vi "SentinelController v33.vi"() -> ()   [LabVIEW 2011] (continued)
                                n3052 = local read "GPIB wait timeout hid"() -> (w2476:u32)
                                n3053 = VISA Open(timeout (0)=w2475, VISA resource name=w2477) -> (VISA resource name=w2474:refnum<visa-resource-name>, error out=w2479:errorcluster)  [unwired: 3 in]
                                n3054 = property class="GPIB Instr"(reference=w2474, error in=w2479, "Timeout"=w2476) -> (error out=w2473:errorcluster)  [unwired: 1 out]
                                n3055 = local write "VISA bus 2 resource name out hid"(w2474) -> ()
                                n3056 = Unbundle By Name(w2473) -> ("status"=w2478:bool)
                                n3057 = local write "VISA bus 2 error out hid"(w2473) -> ()
                                n3058 = local write "VISA bus 2 open error"(w2478) -> ()
                                }
                                frame #1 {
                                n3059 = local write "Exit SC tester H2 StMach hid"(FALSE ("Exit H2 state machine hid")) -> ()
                                n3060 = Concatenate Strings("Bus 2 initializing" ("string"), "\r\n") -> (w2482:string)
                                n3061 = local write "GPIB bus 2 traffic"(w2482) -> ()
                                }
                                frame #2 {
                                n3062 = local write "MT99XX tester states H2 hid"(SC_MT99XX_tester_states."sending *IDN?" ("SC virtual tester states")) -> ()
                                }
                                }
                                }
                                frame "sending *IDN?" {
                                n3063 = flat-sequence {
                                tunnel: [w2494] -> w2487
                                tunnel: [w2493] -> w2486
                                tunnel: w2487 -> [w2508]
                                tunnel: w2486 -> [w2507]
                                tunnel: [w2498] -> w2485
                                tunnel: w2485 -> [w2509]
                                frame #0 {
                                w2488 = "*IDN?"
                                n3064 = local read "VISA bus 2 resource name out hid"() -> (w2497:refnum<visa-resource-name>)
                                n3065 = local read "GPIB bus 2 traffic"() -> (w2492:string)
                                n3066 = local read "VISA bus 2 error out hid"() -> (w2496:errorcluster)
                                n3067 = Concatenate Strings(w2492, "\r\n", "Bus 2 write: " ("string"), w2488) -> (w2490:string)
                                n3068 = VISA Write(VISA resource name=w2497, write buffer=w2488, error in (no error)=w2496) -> (VISA resource name out=w2494:refnum<visa-resource-name>, error out=w2493:errorcluster)  [unwired: 1 out]
                                n3069 = local write "GPIB bus 2 traffic"(w2490) -> ()
                                n3070 = Unbundle By Name(w2493) -> ("status"=w2495:bool)
                                n3071 = local write "GPIB bus 2 write error"(w2495) -> ()
                                }
                                frame #1 {
                                n3072 = local read "GPIB bus 2 traffic"() -> (w2500:string)
                                n3073 = VISA Read(VISA resource name=w2508, byte count=u32 256, error in (no error)=w2507) -> (VISA resource name out=w2505:refnum<visa-resource-name>, read buffer=w2499:string, error out=w2504:errorcluster)  [unwired: 1 out]
                                n3074 = local write "VISA bus 2 resource name out hid"(w2505) -> ()
                                n3075 = Unbundle By Name(w2504) -> ("status"=w2498:bool)
                                n3076 = local write "H2 response to *IDN? hid"(w2499) -> ()
                                n3077 = local write "GPIB bus 2 read error"(w2498) -> ()
                                n3078 = Concatenate Strings(w2500, "\r\n", "Bus 2 read: " ("string"), w2499) -> (w2502:string)
                                n3079 = local write "GPIB bus 2 traffic"(w2502) -> ()
                                }
                                frame #2 {
                                n3080 = case shown="True" w2509 {
                                frame False {
                                n3081 = local write "MT99XX tester states H2 hid"(SC_MT99XX_tester_states."polling *SITES?" ("SC virtual tester states")) -> ()
                                }
                                frame True {
                                n3082 = flat-sequence {
                                frame #0 {
                                n3083 = while {
                                stop <- w2512 stop-if-true
                                n3084 = One Button Dialog(message="Warning:\nVirtual tester does not get a response\nto *IDN? from handler 2.\nCheck GPIB cable and that  handler 2 \nis running and ready to issue a start of test\nby responding with sites ready.", button name ("OK")="Dismiss and retry") -> (true=w2512:bool)
                                n3085 = Wait (ms)(milliseconds to wait=u32 100) -> ()  [unwired: 1 out]
                                }
                                }
                                frame #1 {
                                n3086 = local write "H2 online"(FALSE ("H2 online")) -> ()
                                }
                                frame #2 {
                                n3087 = local write "MT99XX tester states H2 hid"(SC_MT99XX_tester_states."sending *IDN?" ("SC virtual tester states")) -> ()
                                }
                                }
                                }
                                }
                                }
                                }
                                }
                                frame "polling *SITES?" {
                                n3088 = flat-sequence {
                                tunnel: [w2520] -> w2518
                                tunnel: [w2519] -> w2517
                                tunnel: w2518 -> [w2556]
                                tunnel: w2517 -> [w2555]
                                frame #0 {
                                n3089 = while {
                                tunnel: [w2524] -> w2520
                                tunnel: [w2521] -> w2519
                                stop <- w2523 stop-if-true
                                n3090 = stacked-sequence {
                                tunnel: [w2536] -> w2526
                                tunnel: [w2535] -> w2525
                                frame #0 {
                                w2531 = "*SITES?"
                                n3091 = local read "VISA bus 2 resource name out hid"() -> (w2528:refnum<visa-resource-name>)
                                n3092 = local read "VISA bus 2 error out hid"() -> (w2527:errorcluster)
                                n3093 = Concatenate Strings("Handler 2 cycle start" ("string"), "\r\n", "Bus 2 write: " ("string"), w2531) -> (w2533:string)
                                n3094 = VISA Write(VISA resource name=w2528, write buffer=w2531, error in (no error)=w2527) -> (VISA resource name out=w2536:refnum<visa-resource-name>, error out=w2535:errorcluster)  [unwired: 1 out]
                                n3095 = Unbundle By Name(w2535) -> ("status"=w2529:bool)
                                n3096 = local write "GPIB bus 2 traffic"(w2533) -> ()
                                n3097 = local write "GPIB bus 2 write error"(w2529) -> ()
                                }
                                }
                                n3098 = Wait (ms)(milliseconds to wait=u32 1) -> ()  [unwired: 1 out]
                                n3099 = flat-sequence {
                                tunnel: w2526 -> [w2554]
                                tunnel: w2525 -> [w2553]
                                tunnel: [w2540] -> w2524
                                tunnel: [w2538] -> w2523
                                tunnel: [w2537] -> w2521
                                frame #0 {
                                n3100 = local read "GPIB bus 2 traffic"() -> (w2545:string)
                                n3101 = VISA Read(VISA resource name=w2554, byte count=u32 256, error in (no error)=w2553) -> (read buffer=w2540:string, error out=w2551:errorcluster)  [unwired: 2 out]
                                n3102 = Unbundle By Name(w2551) -> ("status"=w2537:bool)
                                n3103 = String Length(string=w2540) -> (length=w2542:i32)
                                n3104 = Scan Value(string=w2540, format string="%b", default (0 dbl)=u8 0) -> (value=w2544:u8)  [unwired: 1 out]
                                n3105 = Concatenate Strings(w2545, "\r\n", "Bus 2 read: " ("string"), w2540) -> (w2547:string)
                                n3106 = local write "GPIB bus 2 read error"(w2537) -> ()
                                n3107 = Greater Than 0?(x=w2542) -> (x > 0?=w2541:bool)
                                n3108 = Greater Than 0?(x=w2544) -> (x > 0?=w2543:bool)
                                n3109 = local write "GPIB bus 2 traffic"(w2547) -> ()
                                n3110 = And(x=w2541, y=w2543) -> (x .and. y?=w2539:bool)
                                n3111 = Or(x=w2539, y=w2537) -> (x .or. y?=w2538:bool)
                                }
                                }
                                }
                                }
                                frame #1 {
                                n3112 = case shown="False" w2555 {
                                tunnel: w2556 -> [w2557 _]
                                frame False {
                                n3113 = flat-sequence {
                                tunnel: w2557 -> [w2558]
                                frame #0 {
                                n3114 = local write "H2 SITES? response hid"(w2558) -> ()
                                n3115 = String Length(string=w2558) -> (length=w2559:i32)
                                n3116 = local write "H2 parallelism"(w2559) -> ()
                                }
                                frame #1 {
                                # "This block adds zeroes (sites not ready)\nto SITES READY from handlers when the\nhandler is running at a lower parallelism\nthan the test program, but has the same\npin mapping for the active sites in common."
                                n3117 = local read "Program Parallelism"() -> (w2561:u32)
                                n3118 = local read "H2 allow lower parallelism"() -> (w2562:bool)
                                n3119 = local read "H2 parallelism"() -> (w2560:u32)
                                n3120 = Less?(x=w2560, y=w2561) -> (x < y?=w2563:bool)
                                n3121 = And(x=w2563, y=w2562) -> (x .and. y?=w2564:bool)
                                n3122 = case shown="False" w2564 {
                                frame False {
                                n3123 = local read "Program Parallelism"() -> (w2567:u32)
                                n3124 = local read "H2 parallelism"() -> (w2565:u32)
                                n3125 = Greater?(x=w2565, y=w2567) -> (0:w2566:bool)
                                n3126 = case shown="True" w2566 {
                                frame False {
                                # "parallelisms must match if arriving here"
                                n3127 = local write "MT99XX tester states H2 hid"(SC_MT99XX_tester_states."testing" ("SC virtual tester states")) -> ()
                                }
                                frame True {
                                n3128 = local write "POWER"(FALSE ("POWER")) -> ()
                                n3129 = local write "MT99XX tester states H2 hid"(SC_MT99XX_tester_states."closing bus" ("SC virtual tester states")) -> ()
                                n3130 = One Button Dialog(message="Fatal error 301:\nTest program cannot support higher\nparallelism on handler 2.\nThe Sentinel Controller program is shutting down.\nPlease correct the mismatch and restart.") -> ()  [unwired: 1 in, 1 out]
                                }
                                }
                                }
                                frame True {
                                n3131 = local read "Program Parallelism"() -> (w2577:u32)
                                n3132 = local read "H2 parallelism"() -> (w2575:u32)
                                n3133 = local read "H2 SITES? response hid"() -> (w2573:string)
                                n3134 = local write "MT99XX tester states H2 hid"(SC_MT99XX_tester_states."testing" ("SC virtual tester states")) -> ()
                                n3135 = Subtract(x=w2577, y=w2575) -> (x-y=w2576:u32)
                                n3136 = for {
                                N: w2576 -> [_]
                                shift-right: [w2578] -> w2572
                                shift-left: w2573 -> [w2579]
                                n3137 = Concatenate Strings(w2579, "0" ("string")) -> (w2578:string)
                                }
                                n3138 = local write "H2 SITES? response hid"(w2572) -> ()
                                }
                                }
                                }
                                frame #2 {
                                n3139 = Tick Count (ms)() -> (millisecond timer value=w2585:u32)
                                n3140 = Tick Count (ms)() -> (millisecond timer value=w2584:u32)
                                n3141 = local write "H2 Ready with sites"(TRUE ("H2 Waiting")) -> ()
                                n3142 = local write "H2 Indexing"(FALSE ("h1 indexing")) -> ()
                                n3143 = local write "H2 Testing"(FALSE ("h1 indexing")) -> ()
                                n3144 = local write "H2 wt start hidden"(w2585) -> ()
                                n3145 = local write "H2 it end hidden"(w2584) -> ()
                                }
                                frame #3 {
                                n3146 = local read "H2 it start hidden"() -> (w2589:u32)
                                n3147 = local read "H2 it end hidden"() -> (w2590:u32)
                                n3148 = Subtract(x=w2590, y=w2589) -> (x-y=w2586:u32)
                                n3149 = local write "MT99XX tester states H2 hid"(SC_MT99XX_tester_states."testing" ("SC virtual tester states")) -> ()
                                n3150 = Divide(x=w2586, y=u32 1000) -> (x/y=w2588:dbl)
                                n3151 = local write "H2 measured  Index Time"(w2588) -> ()
                                }
                                }
                                }
                                frame True {
                                n3152 = flat-sequence {
                                frame #0 {
                                n3153 = local read "VISA bus 2 resource name out hid"() -> (w2595:refnum<visa-resource-name>)
                                n3154 = local read "VISA bus 2 error out hid"() -> (w2594:errorcluster)
                                n3155 = VISA Close(VISA resource name=w2595, error in (no error)=w2594) -> (error out=w2593:errorcluster)
                                n3156 = Unbundle By Name(w2593) -> ("status"=w2592:bool)
                                n3157 = local write "VISA bus 2 close error"(w2592) -> ()
                                }
                                frame #1 {
                                n3158 = local write "VISA bus 2 close error"(FALSE ("VISA bus 1 close error")) -> ()
                                n3159 = Concatenate Strings("Bus 2 error  while reading,\nclosing Bus 2 and re-initializing" ("string"), "\r\n") -> (w2597:string)
                                n3160 = local write "GPIB bus 2 traffic"(w2597) -> ()
                                }
                                frame #2 {
                                n3161 = local write "MT99XX tester states H2 hid"(SC_MT99XX_tester_states."initializing bus" ("SC virtual tester states")) -> ()
                                }
                                }
                                }
                                }
                                }
                                }
                                }
                                frame "testing" {
                                n3162 = flat-sequence {
                                frame #0 {
                                n3163 = while {
                                stop <- w2601 stop-if-true
                                n3164 = local read "H2 Lock"() -> (w2601:bool)
                                n3165 = Wait (ms)(milliseconds to wait=u32 1) -> ()  [unwired: 1 out]
                                }
                                }
                                frame #1 {
                                n3166 = Tick Count (ms)() -> (millisecond timer value=w2613:u32)
                                n3167 = Tick Count (ms)() -> (millisecond timer value=w2612:u32)
                                n3168 = local write "H2 Ready with sites"(FALSE ("waiting")) -> ()
                                n3169 = local write "H2 Indexing"(FALSE ("waiting")) -> ()
                                n3170 = local write "H2 Testing"(TRUE ("testing")) -> ()
                                n3171 = local write "H2 wt end hidden"(w2613) -> ()
                                n3172 = local write "H2 tt start hidden"(w2612) -> ()
                                n3173 = local read "GPIB bus 2 traffic"() -> (w2604:string)
                                n3174 = local write "MT99XX tester states H2 hid"(SC_MT99XX_tester_states."binning" ("SC virtual tester states")) -> ()
                                n3175 = Concatenate Strings(w2604, "\r\n", "Bus 2: " ("string"), "testing" ("string")) -> (w2606:string)
                                n3176 = local write "GPIB bus 2 traffic"(w2606) -> ()
                                }
                                frame #2 {
                                n3177 = local read "H2 wt start hidden"() -> (w2615:u32)
                                n3178 = local read "H2 wt end hidden"() -> (w2614:u32)
                                n3179 = Subtract(x=w2614, y=w2615) -> (x-y=w2618:u32)
                                n3180 = Divide(x=w2618, y=u32 1000) -> (x/y=w2616:dbl)
                                n3181 = local write "H2 measured Wait Time"(w2616) -> ()
                                }
                                frame #3 {
                                n3182 = local write "MT99XX tester states H2 hid"(SC_MT99XX_tester_states."binning" ("MT99XX tester states H2 hid")) -> ()
                                }
                                }
                                }
                                frame "binning" {
                                n3183 = flat-sequence {
                                tunnel: [w2631] -> w2622
                                tunnel: [w2658] -> w2623
                                tunnel: w2622 -> [w2658]
                                tunnel: w2623 -> [w2665]
                                tunnel: [w2664] -> w2621
                                tunnel: [w2663] -> w2620
                                tunnel: w2621 -> [w2716]
                                tunnel: w2620 -> [w2715]
                                frame #0 {
                                n3184 = while {
                                stop <- w2625 continue-if-true
                                n3185 = local read "H2 Lock"() -> (w2625:bool)
                                n3186 = Wait (ms)(milliseconds to wait=u32 1) -> ()  [unwired: 1 out]
                                }
                                }
                                frame #1 {
                                n3187 = local read "Program Parallelism"() -> (w2628:u32)
                                n3188 = local read "H2 parallelism"() -> (w2627:u32)
                                n3189 = local read "H2 allow lower parallelism"() -> (w2629:bool)
                                n3190 = Less?(x=w2627, y=w2628) -> (x < y?=w2630:bool)
                                n3191 = And(x=w2630, y=w2629) -> (x .and. y?=w2626:bool)
                                n3192 = case shown="False" w2626 {
                                tunnel: [w2632 w2643] -> w2631
                                frame False {
                                n3193 = local read "VISA bus 2 resource name out hid"() -> (w2640:refnum<visa-resource-name>)
                                n3194 = local read "Binning string from tester hid"() -> (w2632:string)
                                n3195 = local read "VISA bus 2 error out hid"() -> (w2641:errorcluster)
                                n3196 = local read "GPIB bus 2 traffic"() -> (w2636:string)
                                n3197 = VISA Write(VISA resource name=w2640, write buffer=w2632, error in (no error)=w2641) -> (VISA resource name out=w2638:refnum<visa-resource-name>, error out=w2639:errorcluster)  [unwired: 1 out]
                                n3198 = local write "VISA bus 2 resource name out hid"(w2638) -> ()
                                n3199 = local write "VISA bus 2 error out hid"(w2639) -> ()
                                n3200 = Unbundle By Name(w2639) -> ("status"=w2637:bool)
                                n3201 = Concatenate Strings(w2636, "\r\n", "Bus 2 write: " ("string"), w2632) -> (w2634:string)
                                n3202 = local write "GPIB bus 2 write error"(w2637) -> ()
                                n3203 = local write "GPIB bus 2 traffic"(w2634) -> ()
                                }
                                frame True {
                                n3204 = local read "H2 parallelism"() -> (w2642:u32)
                                n3205 = local read "Binning string from tester hid"() -> (w2644:string)
                                n3206 = local read "VISA bus 2 resource name out hid"() -> (w2655:refnum<visa-resource-name>)
                                n3207 = Multiply(x=w2642, y=u32 8) -> (x*y=w2646:u32)
                                n3208 = local read "VISA bus 2 error out hid"() -> (w2656:errorcluster)
                                n3209 = local read "GPIB bus 2 traffic"() -> (w2651:string)
                                n3210 = Decrement(x=w2646) -> (x-1=w2647:u32)
                                n3211 = String Subset(string=w2644, length (rest)=w2647) -> (substring=w2643:string)  [unwired: 1 in]
                                n3212 = VISA Write(VISA resource name=w2655, write buffer=w2643, error in (no error)=w2656) -> (VISA resource name out=w2653:refnum<visa-resource-name>, error out=w2654:errorcluster)  [unwired: 1 out]
                                n3213 = local write "VISA bus 2 resource name out hid"(w2653) -> ()
                                n3214 = local write "VISA bus 2 error out hid"(w2654) -> ()
                                n3215 = Unbundle By Name(w2654) -> ("status"=w2652:bool)
                                n3216 = Concatenate Strings(w2651, "\r\n", "Bus 2 write: " ("string"), w2643) -> (w2649:string)
                                n3217 = local write "GPIB bus 2 traffic"(w2649) -> ()
                                n3218 = local write "GPIB bus 2 write error"(w2652) -> ()
                                }
                                }
                                }
                                frame #2 {
                                n3219 = Tick Count (ms)() -> (millisecond timer value=w2660:u32)
                                n3220 = Tick Count (ms)() -> (millisecond timer value=w2659:u32)
                                n3221 = local write "H2 Ready with sites"(FALSE ("waiting")) -> ()
                                n3222 = local write "H2 Testing"(FALSE ("waiting")) -> ()
                                n3223 = local write "H2 Indexing"(TRUE ("waiting")) -> ()
                                n3224 = local write "H2 it start hidden"(w2660) -> ()
                                n3225 = local write "H2 tt end hidden"(w2659) -> ()
                                }
                                frame #3 {
                                n3226 = while {
                                tunnel: [w2688] -> w2684 mode=indexing
                                shift-right: [w2689] -> _
                                shift-left: w2665 -> [w2691]
                                stop <- w2686 stop-if-true
                                n3227 = Match Pattern(string=w2691, regular expression=" ") -> (before substring=w2688:string, after substring=w2689:string, offset past match=w2687:i32)  [unwired: 2 out]
                                n3228 = Less Than 0?(x=w2687) -> (x < 0?=w2686:bool)
                                }
                                n3229 = local read "H2 tt start hidden"() -> (w2669:u32)
                                n3230 = local read "H2 tt end hidden"() -> (w2670:u32)
                                n3231 = Subtract(x=w2670, y=w2669) -> (x-y=w2668:u32)
                                n3232 = Divide(x=w2668, y=u32 1000) -> (x/y=w2666:dbl)
                                n3233 = local write "H2 measured Test Time"(w2666) -> ()
                                n3234 = Array Size(array=w2684) -> (size(s)=w2681:i32)
                                n3235 = local read "H2 SITES? response hid"() -> (w2676:string)
                                n3236 = local read "H2 parallelism"() -> (w2675:u32)
                                n3237 = Divide(x=w2681, y=3) -> (x/y=w2683:dbl)
                                n3238 = To Unsigned Byte Integer(number=w2683) -> (unsigned 8bit integer=w2679:u8)
                                n3239 = Not Equal?(x=w2675, y=w2679) -> (x != y?=w2680:bool)
                                n3240 = case shown="True" w2680 {
                                frame False {
                                }
                                frame True {
                                n3241 = One Button Dialog(message="Warning:\nH2 Parallelism Mismatch!\nEither allow this from the system configuration tab\nor change the parallelism on H2. This message will\ncontinue until the problem is corrected.") -> ()  [unwired: 1 in, 1 out]
                                }
                                }
                                n3242 = for {
                                N: w2679 -> [_]
                                tunnel: w2684 -> [w2714]
                                tunnel: w2676 -> [w2705]
                                shift-right: [w2698] -> w2663
                                shift-left: 0 -> [w2697]
                                shift-right: [w2694] -> w2664
                                shift-left: 0 -> [w2692]
                                i -> [w2695]
                                n3243 = Increment(x=w2692) -> (x+1=w2693:i32)
                                n3244 = Increment(x=w2697) -> (x+1=w2696:i32)
                                n3245 = Increment(x=w2695) -> (x+1=w2713:i32)
                                n3246 = String Subset(string=w2705, offset (0)=w2695, length (rest)=1 ("length (rest)")) -> (substring=w2701:string)
                                n3247 = Multiply(x=3, y=w2713) -> (x*y=w2707:i32)
                                n3248 = Equal?(x=w2701, y="1") -> (x = y?=w2699:bool)
                                n3249 = Select(t=w2696, s=w2699, f=w2697) -> (s? t:f=w2698:i32)
                                n3250 = Decrement(x=w2707) -> (x-1=w2706:i32)
                                n3251 = Index Array(array=w2714, index=w2706) -> (element=w2711:string)
                                n3252 = Decimal String To Number(string=w2711, offset=0) -> (number=w2709:i32)  [unwired: 1 in, 1 out]
                                n3253 = Equal?(x=w2709, y=1) -> (x = y?=w2702:bool)
                                n3254 = And(x=w2702, y=w2699) -> (x .and. y?=w2703:bool)
                                n3255 = Select(t=w2693, s=w2703, f=w2692) -> (s? t:f=w2694:i32)
                                }
                                n3256 = local read "H2 Device Count"() -> (w2672:u32)
                                n3257 = local read "H2 Good Units"() -> (w2673:u32)
                                n3258 = Add(x=w2673, y=w2664) -> (x+y=w2674:u32)
                                n3259 = Add(x=w2672, y=w2663) -> (x+y=w2671:u32)
                                n3260 = local write "H2 Good Units"(w2674) -> ()
                                n3261 = local write "H2 Device Count"(w2671) -> ()
                                }
                                frame #4 {
                                n3262 = Divide(x=w2716, y=w2715) -> (x/y=w2717:dbl)
                                n3263 = local read "H2 Device Count"() -> (w2720:u32)
                                n3264 = local read "H2 Good Units"() -> (w2721:u32)
                                n3265 = Multiply(x=w2717, y=100.0) -> (x*y=w2719:dbl)
                                n3266 = local write "H2 cycle yield hid"(w2719) -> ()
                                n3267 = Divide(x=w2721, y=w2720) -> (x/y=w2724:dbl)
                                n3268 = Multiply(x=w2724, y=100.0) -> (x*y=w2722:dbl)
                                n3269 = local write "H2 lot yield mon"(w2722) -> ()
                                }
                                frame #5 {
                                n3270 = local read "H2 online"() -> (w2725:bool)
                                n3271 = local read "POWER"() -> (w2727:bool)
                                n3272 = Compound Arithmetic op=AND(w2725, w2727) -> (w2726:bool)
                                n3273 = case shown="False" w2726 {
                                frame False {
                                n3274 = local write "MT99XX tester states H2 hid"(SC_MT99XX_tester_states."closing bus" ("SC virtual tester states")) -> ()
                                }
                                frame True {
                                n3275 = local write "MT99XX tester states H2 hid"(SC_MT99XX_tester_states."polling *SITES?" ("SC virtual tester states")) -> ()
                                }
                                }
                                }
                                }
                                }
                                frame "closing bus" {
                                n3276 = local read "GPIB bus 2 traffic"() -> (w2734:string)
                                n3277 = local write "Exit SC tester H2 StMach hid"(TRUE ("Exit H2 state machine hid")) -> ()
                                n3278 = local read "VISA bus 2 resource name out hid"() -> (w2738:refnum<visa-resource-name>)
                                n3279 = local read "VISA bus 2 error out hid"() -> (w2737:errorcluster)
                                n3280 = Concatenate Strings(w2734, "\r\n", "Bus 2: closing " ("string")) -> (w2732:string)
                                n3281 = local write "GPIB bus 2 traffic"(w2732) -> ()
                                n3282 = VISA Close(VISA resource name=w2738, error in (no error)=w2737) -> (error out=w2736:errorcluster)
                                n3283 = Unbundle By Name(w2736) -> ("status"=w2735:bool)
                                n3284 = local write "VISA bus 2 close error"(w2735) -> ()
                                }
                              }
                            }
                            frame #1 {
                              n3285 = local read "Slow for  Diagnostics"() -> (w2739:bool)
                              n3286 = case shown="True" w2739 {
                                frame False {
                                }
                                frame True {
                                n3287 = local read "GPIB wait time (ms)"() -> (w2740:u32)
                                n3288 = Wait (ms)(milliseconds to wait=w2740) -> ()  [unwired: 1 out]
                                }
                              }
                            }
                          }
                        }
                        frame "Seiko-Epson NS6040" {
                          n3289 = local write "NS6040 tester states H2 hid"(SC_NS6040_tester_states."initializing bus" ("NS6040 tester states H1 hid")) -> ()
                          n3290 = while {
                            stop <- w2742 stop-if-true
                            n3291 = flat-sequence {
                              frame #0 {
                                n3292 = local read "NS6040 tester states H2 hid"() -> (w2743:T3)
                                n3293 = case shown="\"serial polling handler\"" w2743 {
                                frame "initializing bus", Default {
                                n3294 = flat-sequence {
                                frame #0 {
                                # "bus 2"
                                n3295 = local read "GPIB wait timeout hid"() -> (w2746:u32)
                                n3296 = local read "SentCtrl talks to handler 2 at"() -> (w2748:refnum<visa-resource-name>)
                                n3297 = local read "GPIB wait timeout hid"() -> (w2747:u32)
                                n3298 = VISA Open(timeout (0)=w2746, VISA resource name=w2748) -> (VISA resource name=w2745:refnum<visa-resource-name>, error out=w2750:errorcluster)  [unwired: 3 in]
                                n3299 = property class="GPIB Instr"(reference=w2745, error in=w2750, "Timeout"=w2747) -> (error out=w2744:errorcluster)  [unwired: 1 out]
                                n3300 = local write "VISA bus 2 resource name out hid"(w2745) -> ()
                                n3301 = Unbundle By Name(w2744) -> ("status"=w2749:bool)
                                n3302 = local write "VISA bus 2 error out hid"(w2744) -> ()
                                n3303 = local write "VISA bus 2 open error"(w2749) -> ()
                                }
                                frame #1 {
                                n3304 = local write "Exit SC tester H2 StMach hid"(FALSE ("Exit H2 state machine hid")) -> ()
                                n3305 = Concatenate Strings("Bus 2 initializing" ("string"), "\r\n") -> (w2753:string)
                                n3306 = local write "GPIB bus 2 traffic"(w2753) -> ()
                                }
                                frame #2 {
                                n3307 = local write "NS6040 tester states H2 hid"(SC_NS6040_tester_states."serial polling handler" ("NS6040 tester states H2 hid")) -> ()
                                }
                                }
                                }
                                frame "sending *IDN?" {
                                n3308 = flat-sequence {
                                tunnel: [w2765] -> w2758
                                tunnel: [w2764] -> w2757
                                tunnel: w2758 -> [w2779]
                                tunnel: w2757 -> [w2778]
                                tunnel: [w2769] -> w2756
                                tunnel: w2756 -> [w2780]
                                frame #0 {
                                w2759 = "*IDN?"
                                # "It was discovered that his state is not initialized in application"
                                n3309 = local read "VISA bus 2 resource name out hid"() -> (w2768:refnum<visa-resource-name>)
                                n3310 = local read "GPIB bus 2 traffic"() -> (w2763:string)
                                n3311 = local read "VISA bus 2 error out hid"() -> (w2767:errorcluster)
                                n3312 = Concatenate Strings(w2763, "\r\n", "Bus 2 write: " ("string"), w2759) -> (w2761:string)
                                n3313 = VISA Write(VISA resource name=w2768, write buffer=w2759, error in (no error)=w2767) -> (VISA resource name out=w2765:refnum<visa-resource-name>, error out=w2764:errorcluster)  [unwired: 1 out]
                                n3314 = local write "GPIB bus 2 traffic"(w2761) -> ()
                                n3315 = Unbundle By Name(w2764) -> ("status"=w2766:bool)
                                n3316 = local write "GPIB bus 2 write error"(w2766) -> ()
                                }
                                frame #1 {
                                n3317 = local read "GPIB bus 2 traffic"() -> (w2771:string)
                                n3318 = VISA Read(VISA resource name=w2779, byte count=u32 256, error in (no error)=w2778) -> (VISA resource name out=w2776:refnum<visa-resource-name>, read buffer=w2770:string, error out=w2775:errorcluster)  [unwired: 1 out]
                                n3319 = local write "VISA bus 2 resource name out hid"(w2776) -> ()
                                n3320 = Unbundle By Name(w2775) -> ("status"=w2769:bool)
                                n3321 = local write "H2 response to *IDN? hid"(w2770) -> ()
                                n3322 = local write "GPIB bus 2 read error"(w2769) -> ()
                                n3323 = Concatenate Strings(w2771, "\r\n", "Bus 2 read: " ("string"), w2770) -> (w2773:string)
                                n3324 = local write "GPIB bus 2 traffic"(w2773) -> ()
                                }
                                frame #2 {
                                n3325 = case shown="True" w2780 {
                                frame False {
                                n3326 = local write "NS6040 tester states H2 hid"(SC_NS6040_tester_states."sending FR? " ("NS6040 tester states H2 hid")) -> ()
                                }
                                frame True {
                                n3327 = flat-sequence {
                                frame #0 {
                                n3328 = while {
                                stop <- w2783 stop-if-true
                                n3329 = One Button Dialog(message="Warning:\nVirtual tester does not get a response\nto *IDN? from handler 2.\nCheck GPIB cable and that  handler 2 \nis running and ready to issue a start of test\nby responding with sites ready.", button name ("OK")="Dismiss and retry") -> (true=w2783:bool)
                                n3330 = Wait (ms)(milliseconds to wait=u32 100) -> ()  [unwired: 1 out]
                                }
                                }
                                frame #1 {
                                n3331 = local write "H2 online"(FALSE ("H2 online")) -> ()
                                }
                                frame #2 {
                                n3332 = local write "NS6040 tester states H2 hid"(SC_NS6040_tester_states."sending SRQ MASK" ("NS6040 tester states H2 hid")) -> ()
                                }
                                }
                                }
                                }
                                }
                                }
                                }
                                frame "sending SRQ MASK" {
                                n3333 = flat-sequence {
                                tunnel: [w2789] -> w2788
                                tunnel: w2788 -> [w2798]
                                frame #0 {
                                w2790 = "SRQ MASK 65\n"
                                # "It was discovered that his state is not initialized in application"
                                n3334 = local read "VISA bus 2 resource name out hid"() -> (w2797:refnum<visa-resource-name>)
                                n3335 = local read "VISA bus 2 error out hid"() -> (w2796:errorcluster)
                                n3336 = local read "GPIB bus 2 traffic"() -> (w2794:string)
                                n3337 = VISA Write(VISA resource name=w2797, write buffer=w2790, error in (no error)=w2796) -> (error out=w2795:errorcluster)  [unwired: 2 out]
                                n3338 = Unbundle By Name(w2795) -> ("status"=w2789:bool)
                                n3339 = Concatenate Strings(w2794, "\r\n", "Bus 2 write: " ("string"), w2790) -> (w2792:string)
                                n3340 = local write "GPIB bus 2 write error"(w2789) -> ()
                                n3341 = local write "GPIB bus 2 traffic"(w2792) -> ()
                                }
                                frame #1 {
                                n3342 = case shown="True" w2798 {
                                frame False {
                                n3343 = local write "NS6040 tester states H1 hid"(SC_NS6040_tester_states."serial polling handler" ("NS6040 tester states H1 hid")) -> ()
                                }
                                frame True {
                                n3344 = flat-sequence {
                                frame #0 {
                                n3345 = while {
                                stop <- w2801 stop-if-true
                                n3346 = Wait (ms)(milliseconds to wait=u32 100) -> ()  [unwired: 1 out]
                                n3347 = One Button Dialog(message="Error when writing SRQ MASK to handler 1.\nClosing bus 1.", button name ("OK")="Dismiss and retry") -> (true=w2801:bool)
                                }
                                }
                                frame #1 {
                                n3348 = local write "H1 online"(FALSE ("H1 online")) -> ()
                                }
                                frame #2 {
                                n3349 = local write "NS6040 tester states H1 hid"(SC_NS6040_tester_states."closing bus" ("NS6040 tester states H1 hid")) -> ()
                                }
                                }
                                }
                                }
                                }
                                }
                                }
                                frame "serial polling handler" {
                                w2807 = "1"
                                w2821 = "%08b"  # format string
                                n3350 = flat-sequence {
                                tunnel: [w2828] -> w2822
                                tunnel: [w2827] -> _
                                frame #0 {
                                # "This is a serial poll method that rests the SQR bits after execution"
                                n3351 = local read "VISA bus 2 resource name out hid"() -> (w2829:refnum<visa-resource-name>)
                                n3352 = local read "VISA bus 2 error out hid"() -> (w2830:errorcluster)
                                n3353 = local write "GPIB bus 2 traffic"("Serial polling handler 2") -> ()
                                n3354 = VISA Read STB(8:w2830, 11:w2829) -> (0:w2832:errorcluster, 2:w2828:u16)  [unwired: 1 out]
                                n3355 = Unbundle By Name(w2832) -> ("status"=w2827:bool)
                                n3356 = local write "GPIB bus 2 write error"(w2827) -> ()
                                }
                                }
                                n3357 = Format Into String "Format Into String"(format string=w2821, w2822) -> (resulting string=w2808:string)  [unwired: 2 in, 1 out]
                                n3358 = local read "GPIB bus 2 traffic"() -> (w2820:string)
                                n3359 = String Subset(string=w2808, offset (0)=1, length (rest)=1 ("length (rest)")) -> (substring=w2813:string)
                                n3360 = String Subset(string=w2808, offset (0)=7, length (rest)=1 ("length (rest)")) -> (substring=w2814:string)
                                n3361 = Equal?(x=w2813, y=w2807) -> (x = y?=w2812:bool)
                                n3362 = Equal?(x=w2807, y=w2814) -> (x = y?=w2811:bool)
                                n3363 = Concatenate Strings(w2820, "\r\n", "Bus 2 read: " ("string"), w2808) -> (w2818:string)
                                n3364 = And(x=w2812, y=w2811) -> (x .and. y?=w2806:bool)
                                n3365 = local write "GPIB bus 2 traffic"(w2818) -> ()
                                n3366 = case shown="True" w2806 {
                                frame False {
                                n3367 = flat-sequence {
                                frame #0 {
                                n3368 = Wait (ms)(milliseconds to wait=u32 5) -> ()  [unwired: 1 out]
                                }
                                frame #1 {
                                n3369 = local write "NS6040 tester states H2 hid"(SC_NS6040_tester_states."serial polling handler" ("NS6040 tester states H1 hid")) -> ()
                                }
                                }
                                }
                                frame True {
                                # "This is where the GPIB0 bus controller (PXI Chassis, instrument) has its STB set to 0100 0001 which signals to the tester that a handler is ready with sites"
                                n3370 = flat-sequence {
                                frame #0 {
                                n3371 = local write "H2 Ready with sites"(TRUE ("H2 Waiting")) -> ()
                                }
                                frame #1 {
                                n3372 = local write "NS6040 tester states H1 hid"(SC_NS6040_tester_states."sending Fullsites?" ("NS6040 tester states H1 hid")) -> ()
                                }
                                }
                                }
                                }
                                }
                                frame "sending FR? " {
                                n3373 = while {
                                tunnel: [w2837] -> w2833
                                stop <- w2835 stop-if-true
                                n3374 = flat-sequence {
                                tunnel: [w2847] -> w2841
                                tunnel: [w2846] -> w2840
                                tunnel: w2841 -> [w2851]
                                tunnel: w2840 -> [w2850]
                                tunnel: [w2849] -> w2837
                                tunnel: [w2848] -> w2836
                                frame #0 {
                                w2842 = "FR?"
                                # "It was discovered that his state is not initialized in application"
                                n3375 = local read "VISA bus 2 resource name out hid"() -> (w2845:refnum<visa-resource-name>)
                                n3376 = local read "VISA bus 2 error out hid"() -> (w2844:errorcluster)
                                n3377 = local write "GPIB bus 2 traffic"(w2842) -> ()
                                n3378 = VISA Write(VISA resource name=w2845, write buffer=w2842, error in (no error)=w2844) -> (VISA resource name out=w2847:refnum<visa-resource-name>, error out=w2846:errorcluster)  [unwired: 1 out]
                                n3379 = Unbundle By Name(w2846) -> ("status"=w2843:bool)
                                n3380 = local write "GPIB bus 2 write error"(w2843) -> ()
                                }
                                frame #1 {
                                n3381 = local read "GPIB bus 2 traffic"() -> (w2857:string)
                                n3382 = VISA Read(VISA resource name=w2851, byte count=u32 256, error in (no error)=w2850) -> (VISA resource name out=w2858:refnum<visa-resource-name>, read buffer=w2848:string, error out=w2853:errorcluster)  [unwired: 1 out]
                                n3383 = local write "VISA bus 2 resource name out hid"(w2858) -> ()
                                n3384 = local write "H2 response to FR? hid"(w2848) -> ()
                                n3385 = Unbundle By Name(w2853) -> ("status"=w2849:bool)
                                n3386 = local write "GPIB bus 2 write error"(w2849) -> ()
                                n3387 = Concatenate Strings(w2857, "\r\n", "Bus 2 read: " ("string"), w2848) -> (w2855:string)
                                n3388 = local write "GPIB bus 2 traffic"(w2855) -> ()
                                }
                                }
                                n3389 = Equal?(x=w2836, y="FR0") -> (x = y?=w2838:bool)
                                n3390 = Or(x=w2838, y=w2837) -> (x .or. y?=w2835:bool)
                                n3391 = Wait (ms)(milliseconds to wait=u32 20) -> ()  [unwired: 1 out]
                                }
                                n3392 = case shown="False" w2833 {
                                frame False {
                                n3393 = local write "NS6040 tester states H2 hid"(SC_NS6040_tester_states."sending Fullsites?" ("NS6040 tester states H1 hid")) -> ()
                                }
                                frame True {
                                n3394 = flat-sequence {
                                frame #0 {
                                n3395 = while {
                                stop <- w2860 stop-if-true
                                n3396 = Wait (ms)(milliseconds to wait=u32 100) -> ()  [unwired: 1 out]
                                n3397 = One Button Dialog(message="Read error while reading FR?,\nclosing Bus and re-initializing" ("Reply from Sentinel Controller to tester")) -> (true=w2860:bool)  [unwired: 1 in]
                                }
                                }
                                frame #1 {
                                n3398 = local read "VISA bus 2 resource name out hid"() -> (w2866:refnum<visa-resource-name>)
                                n3399 = local read "VISA bus 2 error out hid"() -> (w2865:errorcluster)
                                n3400 = VISA Close(VISA resource name=w2866, error in (no error)=w2865) -> (error out=w2864:errorcluster)
                                n3401 = Unbundle By Name(w2864) -> ("status"=w2863:bool)
                                n3402 = local write "VISA bus 2 close error"(w2863) -> ()
                                }
                                frame #2 {
                                n3403 = local write "VISA bus 2 close error"(FALSE ("H1 online")) -> ()
                                n3404 = local write "NS6040 tester states H2 hid"(SC_NS6040_tester_states."initializing bus" ("NS6040 tester states H1 hid")) -> ()
                                }
                                }
                                }
                                }
                                }
                                frame "sending Fullsites?" {
                                n3405 = flat-sequence {
                                frame #0 {
                                n3406 = flat-sequence {
                                tunnel: [w2874] -> w2872
                                tunnel: [w2873] -> w2871
                                tunnel: w2872 -> [w2881]
                                tunnel: w2871 -> [w2880]
                                tunnel: [w2881] -> w2870
                                tunnel: [w2880] -> w2869
                                tunnel: w2870 -> [w2883]
                                tunnel: w2869 -> [w2882]
                                frame #0 {
                                w2876 = "FULLSITES?"
                                n3407 = local read "VISA bus 2 resource name out hid"() -> (w2875:refnum<visa-resource-name>)
                                n3408 = local read "VISA bus 2 error out hid"() -> (w2877:errorcluster)
                                n3409 = local write "GPIB bus 2 traffic"(w2876) -> ()
                                n3410 = VISA Write(VISA resource name=w2875, write buffer=w2876, error in (no error)=w2877) -> (VISA resource name out=w2874:refnum<visa-resource-name>, error out=w2873:errorcluster)  [unwired: 1 out]
                                n3411 = Unbundle By Name(w2873) -> ("status"=w2878:bool)
                                n3412 = local write "GPIB bus 2 write error"(w2878) -> ()
                                }
                                frame #1 {
                                n3413 = Wait (ms)(milliseconds to wait=u32 2) -> ()  [unwired: 1 out]
                                }
                                frame #2 {
                                n3414 = local read "GPIB bus 2 traffic"() -> (w2890:string)
                                n3415 = VISA Read(VISA resource name=w2883, byte count=u32 256, error in (no error)=w2882) -> (VISA resource name out=w2888:refnum<visa-resource-name>, read buffer=w2891:string, error out=w2885:errorcluster)  [unwired: 1 out]
                                n3416 = local write "VISA bus 2 resource name out hid"(w2888) -> ()
                                n3417 = local write "H2 FULLSITES? response hid"(w2891) -> ()
                                n3418 = Unbundle By Name(w2885) -> ("status"=w2892:bool)
                                n3419 = Concatenate Strings(w2890, "\r\n", "Bus 2 read: " ("string"), w2891) -> (w2889:string)
                                n3420 = local write "GPIB bus 2 read error"(w2892) -> ()
                                n3421 = local write "GPIB bus 2 traffic"(w2889) -> ()
                                }
                                }
                                }
                                frame #1 {
                                n3422 = local read "GPIB bus 2 read error"() -> (w2893:bool)
                                n3423 = case shown="False" w2893 {
                                frame False {
                                n3424 = flat-sequence {
                                frame #0 {
                                w2902 = "%032b"  # format string
                                n3425 = local read "H2 FULLSITES? response hid"() -> (w2895:string)
                                n3426 = call <vilib>:"Space Constant.vi"() -> ("String"=w2897:string)
                                n3427 = Concatenate Strings("Fullsites?\n" ("regular expression"), w2897) -> (w2896:string)
                                n3428 = call <vilib>:"Trim Whitespace.vi"("string"=w2895) -> ("trimmed string"=w2894:string)  [unwired: 1 in]
                                n3429 = Match Pattern(string=w2894, regular expression=w2896) -> (after substring=w2900:string)  [unwired: 1 in, 3 out]
                                n3430 = Hexadecimal String To Number(string=w2900, default (0uL)=u64 0 ("default (0 U32)")) -> (number=w2903:u64)  [unwired: 1 in, 1 out]
                                n3431 = Format Into String "Format Into String"(format string=w2902, w2903) -> (resulting string=w2899:string)  [unwired: 2 in, 1 out]
                                n3432 = local write "H2 FULLSITES? binary hid"(w2899) -> ()
                                }
                                frame #1 {
                                n3433 = Tick Count (ms)() -> (millisecond timer value=w2907:u32)
                                n3434 = Tick Count (ms)() -> (millisecond timer value=w2906:u32)
                                n3435 = local write "H2 Indexing"(FALSE ("h1 indexing")) -> ()
                                n3436 = local write "H2 Testing"(FALSE ("h1 indexing")) -> ()
                                n3437 = local write "H2 wt start hidden"(w2907) -> ()
                                n3438 = local write "H2 it end hidden"(w2906) -> ()
                                }
                                frame #2 {
                                n3439 = local read "H2 it start hidden"() -> (w2911:u32)
                                n3440 = local read "H2 it end hidden"() -> (w2912:u32)
                                n3441 = Subtract(x=w2912, y=w2911) -> (x-y=w2908:u32)
                                n3442 = Divide(x=w2908, y=u32 1000) -> (x/y=w2910:dbl)
                                n3443 = local write "H2 measured  Index Time"(w2910) -> ()
                                }
                                frame #3 {
                                n3444 = local write "NS6040 tester states H2 hid"(SC_NS6040_tester_states."testing" ("NS6040 tester states H1 hid")) -> ()
                                }
                                }
                                }
                                frame True {
                                n3445 = flat-sequence {
                                frame #0 {
                                n3446 = while {
                                stop <- w2914 stop-if-true
                                n3447 = Wait (ms)(milliseconds to wait=u32 100) -> ()  [unwired: 1 out]
                                n3448 = One Button Dialog(message="Read error while reading FULLSITES?,\nclosing Bus and re-initializing" ("Reply from Sentinel Controller to tester")) -> (true=w2914:bool)  [unwired: 1 in]
                                }
                                }
                                frame #1 {
                                n3449 = local read "VISA bus 2 resource name out hid"() -> (w2917:refnum<visa-resource-name>)
                                n3450 = local read "VISA bus 2 error out hid"() -> (w2918:errorcluster)
                                n3451 = VISA Close(VISA resource name=w2917, error in (no error)=w2918) -> (error out=w2920:errorcluster)
                                n3452 = Unbundle By Name(w2920) -> ("status"=w2919:bool)
                                n3453 = local write "VISA bus 2 close error"(w2919) -> ()
                                }
                                frame #2 {
                                n3454 = local write "VISA bus 2 close error"(FALSE ("H1 online")) -> ()
                                n3455 = local write "NS6040 tester states H2 hid"(SC_NS6040_tester_states."initializing bus" ("NS6040 tester states H1 hid")) -> ()
                                }
                                }
                                }
                                }
                                }
                                }
                                }
                                frame "testing" {
                                n3456 = flat-sequence {
                                frame #0 {
                                n3457 = while {
                                stop <- w2923 stop-if-true
                                n3458 = local read "H2 Lock"() -> (w2923:bool)
                                n3459 = Wait (ms)(milliseconds to wait=u32 1) -> ()  [unwired: 1 out]
                                }
                                }
                                frame #1 {
                                n3460 = Tick Count (ms)() -> (millisecond timer value=w2934:u32)
                                n3461 = Tick Count (ms)() -> (millisecond timer value=w2933:u32)
                                n3462 = local write "H2 Ready with sites"(FALSE ("waiting")) -> ()
                                n3463 = local write "H2 Indexing"(FALSE ("waiting")) -> ()
                                n3464 = local write "H2 Testing"(TRUE ("testing")) -> ()
                                n3465 = local write "H2 wt end hidden"(w2934) -> ()
                                n3466 = local write "H2 tt start hidden"(w2933) -> ()
                                n3467 = local read "GPIB bus 2 traffic"() -> (w2926:string)
                                n3468 = Concatenate Strings(w2926, "\r\n", "Bus 2: " ("string"), "testing" ("string")) -> (w2928:string)
                                n3469 = local write "GPIB bus 2 traffic"(w2928) -> ()
                                }
                                frame #2 {
                                n3470 = local read "H2 wt start hidden"() -> (w2936:u32)
                                n3471 = local read "H2 wt end hidden"() -> (w2935:u32)
                                n3472 = Subtract(x=w2935, y=w2936) -> (x-y=w2939:u32)
                                n3473 = Divide(x=w2939, y=u32 1000) -> (x/y=w2937:dbl)
                                n3474 = local write "H2 measured Wait Time"(w2937) -> ()
                                }
                                frame #3 {
                                n3475 = local write "NS6040 tester states H2 hid"(SC_NS6040_tester_states."sending BINON?" ("NS6040 tester states H1 hid")) -> ()
                                }
                                }
                                }
                                frame "sending BINON?" {
                                n3476 = flat-sequence {
                                tunnel: [w2948] -> w2943
                                tunnel: [w2947] -> w2942
                                tunnel: w2943 -> [w2959]
                                tunnel: w2942 -> [w2958]
                                tunnel: [w2957] -> w2941
                                tunnel: w2941 -> [w2975]
                                frame #0 {
                                n3477 = while {
                                stop <- w2945 continue-if-true
                                n3478 = local read "H2 Lock"() -> (w2945:bool)
                                n3479 = Wait (ms)(milliseconds to wait=u32 1) -> ()  [unwired: 1 out]
                                }
                                }
                                frame #1 {
                                n3480 = local read "Binning string from tester hid"() -> (w2946:string)
